vi "Create.vi"(8 "error in (no error)":errorcluster, 11 "TemplatePlugin in":refnum<class "TemplatePlugin.lvclass">) -> (0 "error out":errorcluster, 3 "TemplatePlugin out":refnum<class "TemplatePlugin.lvclass">)   [LabVIEW 2021, in "TemplatePlugin.lvclass"]
uses:
  TemplatePlugin.lvclass
  D:/dev/CIF-LVCore/src/CIFCore/Class/CIFCorePlugin.lvclass
  <vilib>/CIF Foundation/CIF Channels Core/CIFChannels/CIFChannels.lvclass
  CIF-LVCore/src/CIFCore/Class/CIFCorePlugin.lvclass/CIFCorePlugin.ctl
  <vilib>/CIF Foundation/CIF Channels Core/CIFChannels/CIFChannels.lvclass/CIFChannels.ctl
  CIF-LVCore/src/Channels/CIFChannelMng/CIFChannelMng.lvclass/CIFChannelMng.ctl
  <vilib>/CIF Foundation/CIF Channels Core/CIFChannels/Accessors/Read Name.vi
  <vilib>/CIF Foundation/CIF Channels Core/CIFChannels/Accessors/Read Custom Config Data.vi
  <vilib>/CIF Foundation/CIF Channels Core/CIFChannels/Accessors/Read Type.vi
  <vilib>/CIF Foundation/CIF Channels Core/CIFChannels/Accessors/Read Pattern.vi
  <vilib>/CIF Foundation/CIF Channels Core/CIFChannels/Accessors/Read Direction.vi
  <vilib>/CIF Foundation/CIF Channels Core/CIFChannels/Accessors/Read Channel State.vi
  <vilib>/CIF Foundation/CIF Channels Core/ChannelCommon/Utilities/Add Error.vi
  <vilib>/CIF Foundation/CIF Utilities/Errors/Append Error Location.vi
  Common/TemplateCommon.lvlib
  CIF-LVCore/src/CIFCore/Class/CIFCorePlugin.lvclass
  CIF-LVCore/src/CIFCore/Common/Typedef/Timing Overrides.ctl
  CIF-LVCore/src/CIFCore/Common/CIFCoreCommon.lvlib
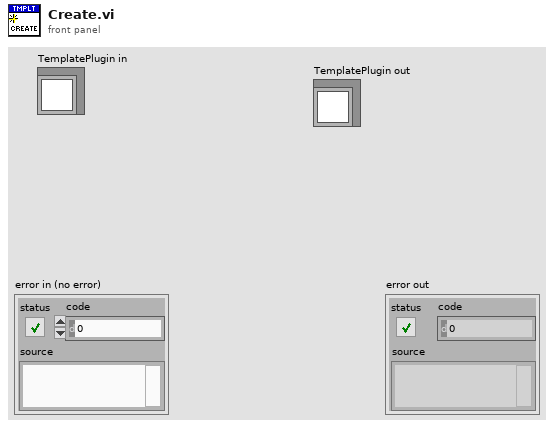
[diagram p1: front panel]
types:
  T1 = typedef "CIFCoreCommon.lvlib/Timing Overrides.ctl" = cluster{"Override Timing":bool, "Skip Sleep":bool, "Period (s)":dbl}
  T2 = typedef "ChannelRegistrar.lvlib/Channel Definition.ctl" = cluster{"Name":string, "Direction":T3, "Type":T4, "Custom Config Data":u8[]}
  T3 = typedef "CIFChannels.lvclass/Direction.ctl" = enum16{"Publisher", "Subscriber"}
  T4 = typedef "ChannelRegistrar.lvlib/Registered Channel Types.ctl" = enum16{"Custom", "Double_Tag", "I64_Tag", "U64_Tag", "U8_FIFO", "CAN_FIFO", "L2Enet_FIFO", "DAQ_FIFO", "Universal_FIFO", "String_Tag"}
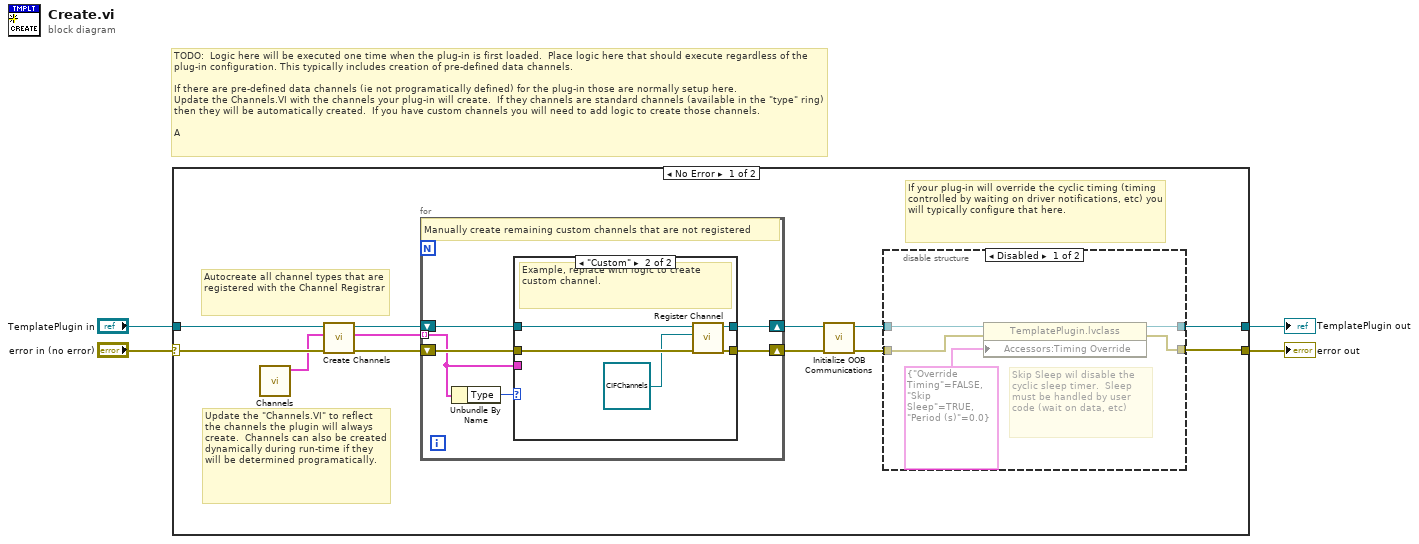
[diagram p0: block diagram]
diagram:
  # "TODO:  Logic here will be executed one time when the plug-in is first loaded.  Place logic here that should execute regardless of the plug-in configuration. This typically includes creation of pre-defined data channels.\n\nIf there are pre-defined data channels (ie not programatically defined) for the plug-in those are normally setup here.  \nUpdate the Channels.VI with the channels your plug-in will create.  If they channels are standard channels (available in the \"type\" ring) then they will be automatically created.  If you have custom channels you will need to add logic to create those channels.\n\nA"
  n1 = case shown="No Error" "error in (no error)" {
    selector: "error in (no error)" -> [w15 w38]
    tunnel: [w9 w38] -> w1
    tunnel: [w10 w37] -> w2
    tunnel: "TemplatePlugin in" -> [w16 w37]
    frame No Error {
      # "If your plug-in will override the cyclic timing (timing controlled by waiting on driver notifications, etc) you will typically configure that here."
      # "Update the \"Channels.VI\" to reflect the channels the plugin will always create.  Channels can also be created dynamically during run-time if they will be determined programatically."
      # "Autocreate all channel types that are registered with the Channel Registrar"
      n2 = call "Channels.vi"() -> ("Channels to Create"=w14:T2[])  [unwired: 10 in, 1 out]
      n3 = call "Create Channels.vi"("error in (no error)"=w15, "Channels to Create in"=w14, "CIFCorePlugin in"=w16) -> ("error out"=w11:errorcluster, "Channels to Create out"=w13:T2[], "CIFCorePlugin out"=w12:refnum<class "TemplatePlugin.lvclass">)  [unwired: 6 in]
      n4 = for {
        tunnel: w13 -> [w24] mode=indexing
        shift-right: [w27] -> w8
        shift-left: w12 -> [w29]
        shift-right: [w26] -> w7
        shift-left: w11 -> [w28]
        # "Manually create remaining custom channels that are not registered"
        n5 = Unbundle By Name(w24) -> ("Type"=w25:T4)
        n6 = case shown="\"Custom\"" w25 {
          tunnel: w29 -> [w31 w36]
          tunnel: w28 -> [w30 w35]
          tunnel: [w31 w34] -> w27
          tunnel: [w30 w33] -> w26
          tunnel: w24 -> [_ _]
          frame Default {
          }
          frame "Custom" {
            # "Example, replace with logic to create custom channel."
            n7 = call "Register Channel.vi"("error in (no error)"=w35, "Channel"=refnum<class "CIFChannels.lvclass"> refnum, "CIFCorePlugin in"=w36) -> ("error out"=w33:errorcluster, "CIFCorePlugin out"=w34:refnum<class "TemplatePlugin.lvclass">)  [unwired: 7 in]
          }
        }
      }
      n8 = call "Initialize OOB Communications.vi"("error in (no error)"=w7, "CIFTemplatePlugin in"=w8) -> ("error out"=w5:errorcluster, "CIFTemplatePlugin out"=w6:refnum<class "TemplatePlugin.lvclass">)  [unwired: 8 in]
      n9 = disable-structure shown="Disabled" {
        disable-tunnel: w6 -> [w21 w23]
        disable-tunnel: w5 -> [w20 w22]
        disable-tunnel: [w19 w23] -> w10
        disable-tunnel: [w18 w22] -> w9
        frame Disabled {
          # "Skip Sleep wil disable the cyclic sleep timer.  Sleep must be handled by user code (wait on data, etc)"
          n10 = property class="TemplatePlugin.lvclass"(reference=w21, error in=w20, "Accessors:Timing Override"=T1 {"Override Timing"=FALSE, "Skip Sleep"=TRUE, "Period (s)"=0.0} ("Timing Override")) -> (reference out=w19:refnum<class "TemplatePlugin.lvclass">, error out=w18:errorcluster)
        }
        frame Enabled {
        }
      }
    }
    frame Error {
    }
  }
  "TemplatePlugin out" <- w2
  "error out" <- w1
